vi "GetStructureDiagrams.vi"(5 "Structure in":refnum<class "Structure.lvclass">, 6 "error in":errorcluster, 9 "VI Interpreter in":refnum<class "VI Interpreter.lvclass">) -> (0 "error out":errorcluster, 3 "VI Interpreter out":refnum<class "VI Interpreter.lvclass">, 4 "Structure out":refnum<class "Structure.lvclass">)   [LabVIEW 2014, in "Raspberry Pi Compatible Compiler for LabVIEW.lvlib" / "VI Interpreter.lvclass"]
uses:
  VI Interpreter.lvclass
  Structure/Structure.lvclass
  Diagram/Diagram.lvclass/Diagram.ctl
  Structure/Structure.lvclass/Structure.ctl
  Diagram/Diagram.lvclass
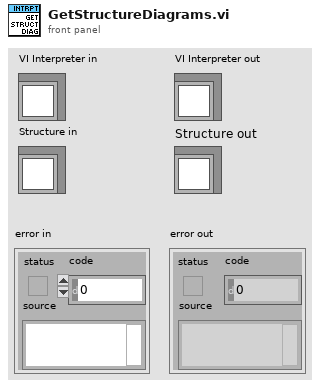
[diagram p1: front panel]
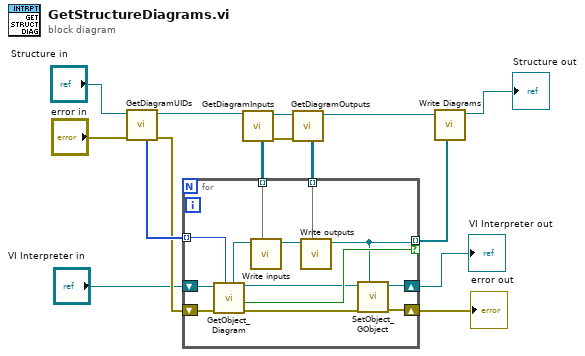
[diagram p0: block diagram]
diagram:
  n1 = call-dynamic "GetDiagramUIDs.vi"("error in"="error in", "Structure in"="Structure in") -> ("error out"=w14:errorcluster, "Structure out"=w6:refnum<class "Structure.lvclass">, "diagrams"=w15:i32[])  [unwired: 5 in]
  n2 = call-dynamic "GetDiagramInputs.vi"("Structure in"=w6) -> ("error out"=w3:errorcluster, "Structure out"=w4:refnum<class "Structure.lvclass">, "inputs terminals"=w5:refnum<class "Terminal.lvclass">[][])  [unwired: 6 in]
  n3 = call-dynamic "GetDiagramOutputs.vi"("error in"=w3, "Structure in"=w4) -> ("Structure out"=w1:refnum<class "Structure.lvclass">, "output terminals"=w2:refnum<class "Terminal.lvclass">[][])  [unwired: 5 in, 1 out]
  n4 = for {
    shift-right: [w20] -> w13
    shift-left: "VI Interpreter in" -> [w28]
    tunnel: w15 -> [w27] mode=indexing
    shift-right: [w19] -> w12
    shift-left: w14 -> [w26]
    tunnel: [w16] -> w8 mode=indexing if=w25
    tunnel: w5 -> [w22] mode=indexing
    tunnel: w2 -> [w21] mode=indexing
    n5 = call "GetObject_Diagram.vi"("UID"=w27, "error in"=w26, "VI Interpreter in"=w28) -> ("error out"=w18:errorcluster, "found"=w25:bool, "VI Interpreter out"=w17:refnum<class "VI Interpreter.lvclass">, "Diagram"=w24:refnum<class "Diagram.lvclass">)  [unwired: 3 in]
    n6 = call "Write inputs.vi"("inputs"=w22, "Diagram in"=w24) -> ("Diagram out"=w23:refnum<class "Diagram.lvclass">)  [unwired: 7 in]
    n7 = call "Write outputs.vi"("outputs"=w21, "Diagram in"=w23) -> ("Diagram out"=w16:refnum<class "Diagram.lvclass">)  [unwired: 7 in]
    n8 = call "SetObject_GObject.vi"("GObject"=w16, "error in"=w18, "VI Interpreter in"=w17) -> ("error out"=w19:errorcluster, "VI Interpreter out"=w20:refnum<class "VI Interpreter.lvclass">)  [unwired: 5 in]
  }
  "error out" <- w12
  "VI Interpreter out" <- w13
  n9 = call "Write Diagrams.vi"("Diagrams"=w8, "Structure in"=w1) -> ("Structure out"=→"Structure out":refnum<class "Structure.lvclass">)  [unwired: 7 in]
